vi "Update State Data.vi"(8 "error in (no error)":errorcluster, 9 "Data":variant, 10 "Argument":string, 11 "State Data":T1) -> (0 "error out":errorcluster, 3 "State Data out":T1)   [LabVIEW 2020, in "MacroAssert.lvlib"]
doc: "Updates one or more elements of <B>State Data</B> based on <B>Argument</B> and <B>Data</B>."
uses:
  MacroAssert.lvlib
  CTLs/State Data.ctl
  Classes/Macro/Macro.lvclass
  CTLs/Refs.ctl
  CTLs/Report Data.ctl
  CTLs/Config.ctl
  <vilib>/Utility/error.llb/Error Cluster From Error Code.vi
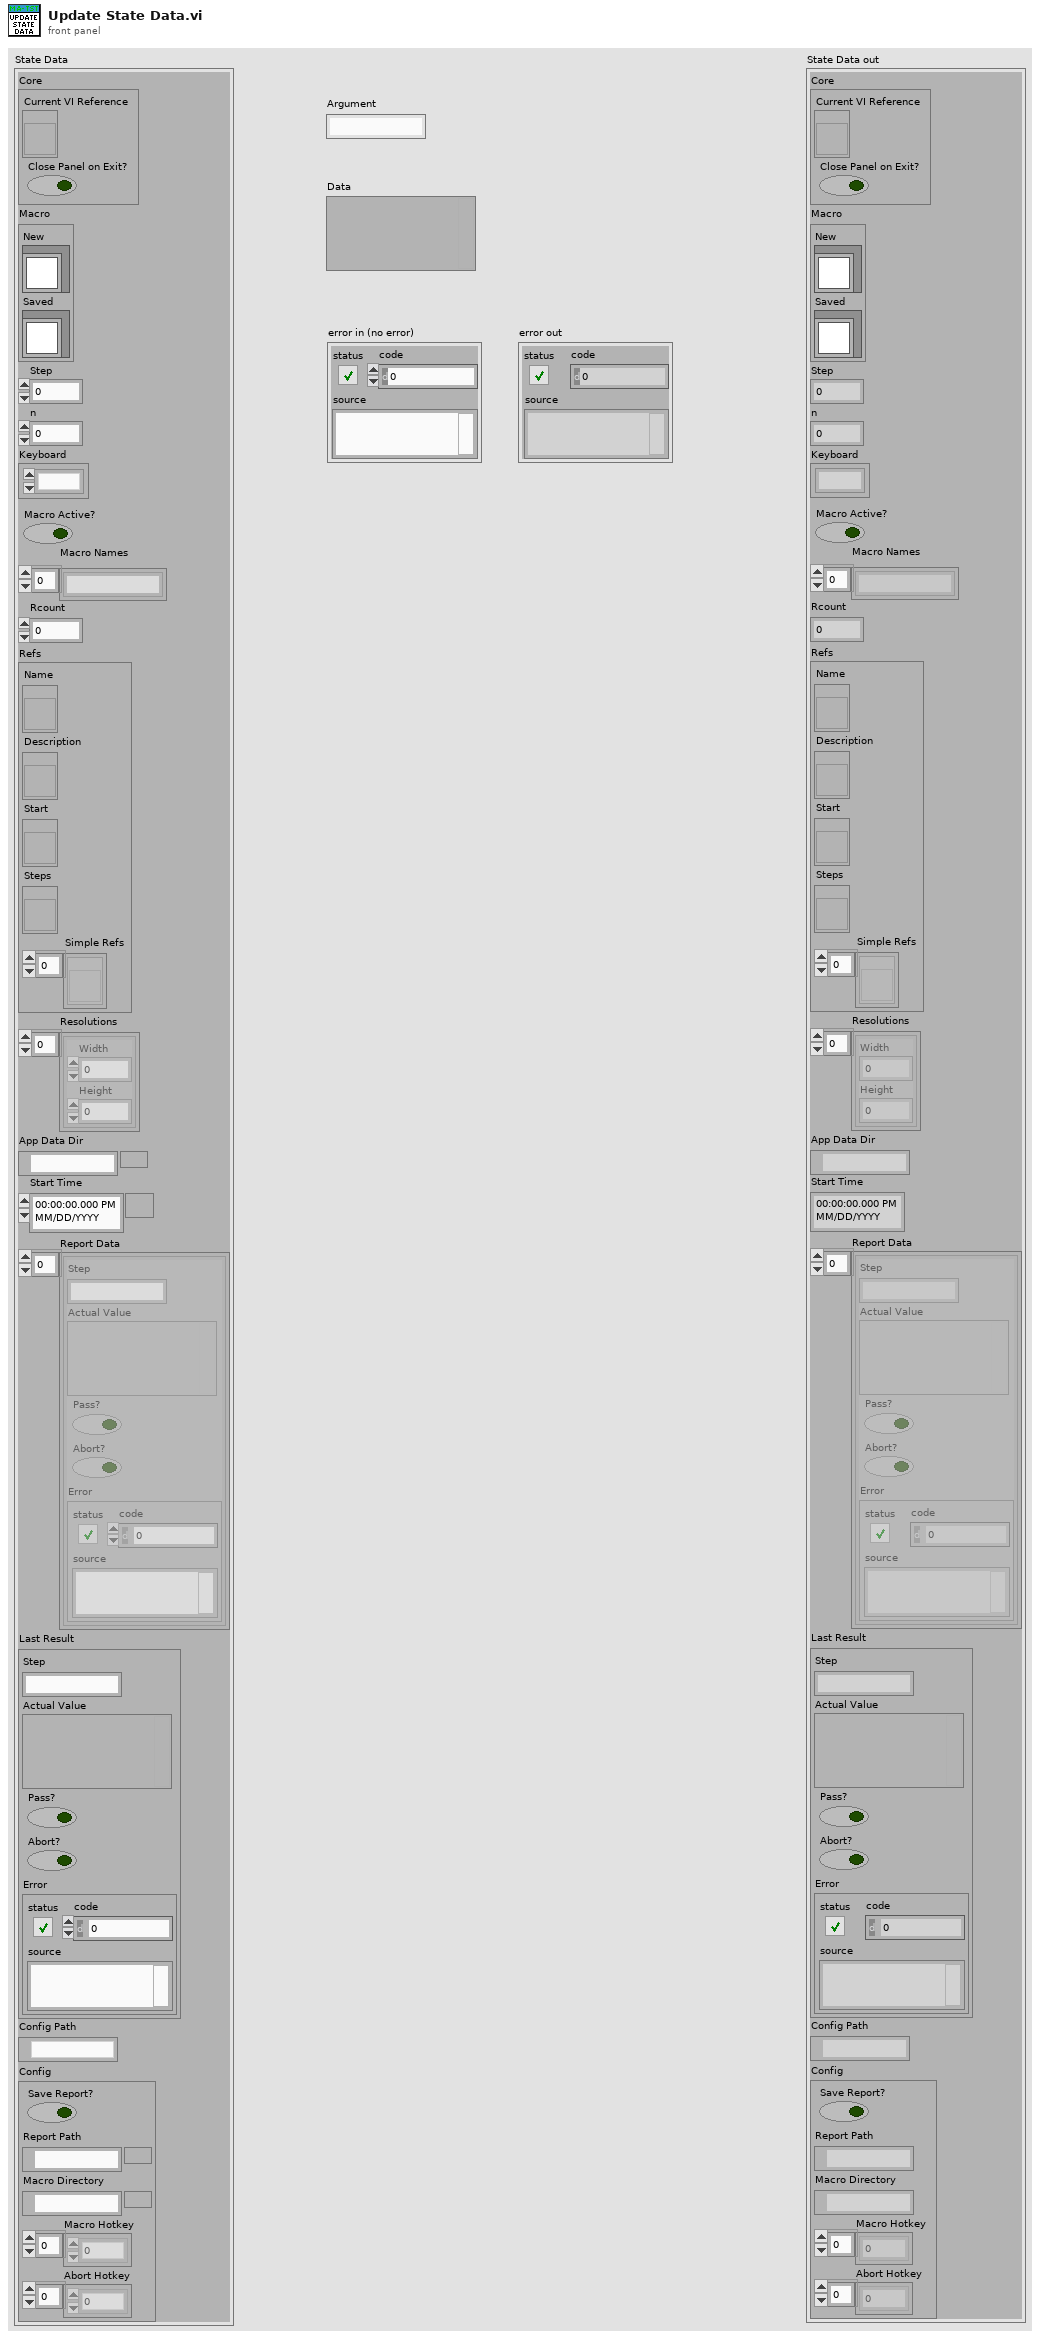
[diagram p1: front panel]
types:
  T1 = typedef "MacroAssert.lvlib/State Data.ctl" = cluster{"Core":cluster{"Current VI Reference":refnum<vi>, "Close Panel on Exit?":bool}, "Macro":cluster{"New":refnum<class "Macro.lvclass">, "Saved":refnum<class "Macro.lvclass">}, "Step":i32, "n":i32, "Keyboard":refnum<k1>, "Macro Active?":bool, "Macro Names":string[], "Rcount":i32, "Refs":T2, "Resolutions":cluster{"Width":i16, "Height":i16}[], "App Data Dir":path, "Start Time":timestamp, "Report Data":T3[], "Last Result":T3, "Config Path":path, "Config":T4}
  T2 = typedef "MacroAssert.lvlib/Refs.ctl" = cluster{"Name":refnum<vi>, "Description":refnum<vi>, "Start":refnum<vi>, "Steps":refnum<vi>, "Simple Refs":refnum<vi>[]}
  T3 = typedef "MacroAssert.lvlib/Report Data.ctl" = cluster{"Step":string, "Actual Value":variant, "Pass?":bool, "Abort?":bool, "Error":errorcluster}
  T4 = typedef "MacroAssert.lvlib/Config.ctl" = cluster{"Save Report?":bool, "Report Path":path, "Macro Directory":path, "Macro Hotkey":enum16{"0", "1", "2", "3", "4", "5", "6", "7", "8", "9", "A", "B", "C", "D", "E", "F", "G", "H", "I", "J", "K", "L", "M", "N", "O", "P", "Q", "R", "S", "T", "U", "V", "W", "X", "Y", "Z", "F1", "F2", "F3", "F4", "F5", "F6", "F7", "F8", "F9", "F10", "F11", "F12", "F13", "F14", "F15", "ADD", "BACK", "BACKSLASH", "CAPITAL", "COMMA", "DECIMAL", "DELETE", "DIVIDE", "DOWN", "END", "EQUALS", "ESCAPE", "GRAVE (`)", "HOME", "INSERT", "LBRACKET", "LCONTROL", "LEFT", "L ALT", "LSHIFT", "LWIN", "MINUS", "MULTIPLY", "NEXT", "NUMLOCK", "NUMPAD_0", "NUMPAD_1", "NUMPAD_2", "NUMPAD_3", "NUMPAD_4", "NUMPAD_5", "NUMPAD_6", "NUMPAD_7", "NUMPAD_8", "NUMPAD_9", "PAUSE", "PERIOD", "PRIOR (PG UP)", "RBRACKET", "RCONTROL", "RETURN", "RIGHT", "R ALT", "RSHIFT", "RWIN", "SCROLL", "SEMICOLON", "SLASH", "SPACE", "SUBTRACT", "TAB", "UP", "ENTER (num pad)", "' (quote)"}[], "Abort Hotkey":enum16{"0", "1", "2", "3", "4", "5", "6", "7", "8", "9", "A", "B", "C", "D", "E", "F", "G", "H", "I", "J", "K", "L", "M", "N", "O", "P", "Q", "R", "S", "T", "U", "V", "W", "X", "Y", "Z", "F1", "F2", "F3", "F4", "F5", "F6", "F7", "F8", "F9", "F10", "F11", "F12", "F13", "F14", "F15", "ADD", "BACK", "BACKSLASH", "CAPITAL", "COMMA", "DECIMAL", "DELETE", "DIVIDE", "DOWN", "END", "EQUALS", "ESCAPE", "GRAVE (`)", "HOME", "INSERT", "LBRACKET", "LCONTROL", "LEFT", "L ALT", "LSHIFT", "LWIN", "MINUS", "MULTIPLY", "NEXT", "NUMLOCK", "NUMPAD_0", "NUMPAD_1", "NUMPAD_2", "NUMPAD_3", "NUMPAD_4", "NUMPAD_5", "NUMPAD_6", "NUMPAD_7", "NUMPAD_8", "NUMPAD_9", "PAUSE", "PERIOD", "PRIOR (PG UP)", "RBRACKET", "RCONTROL", "RETURN", "RIGHT", "R ALT", "RSHIFT", "RWIN", "SCROLL", "SEMICOLON", "SLASH", "SPACE", "SUBTRACT", "TAB", "UP", "ENTER (num pad)", "' (quote)"}[]}
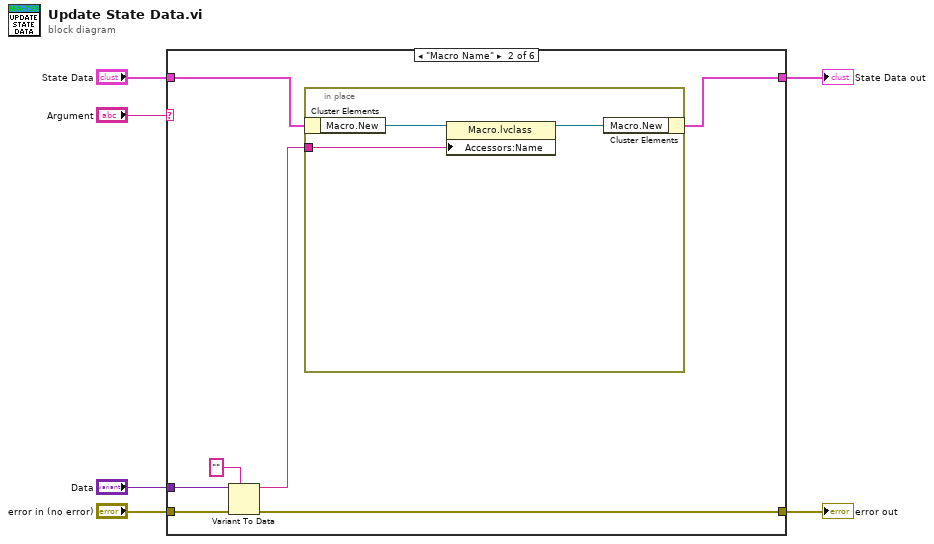
[diagram p0: block diagram]
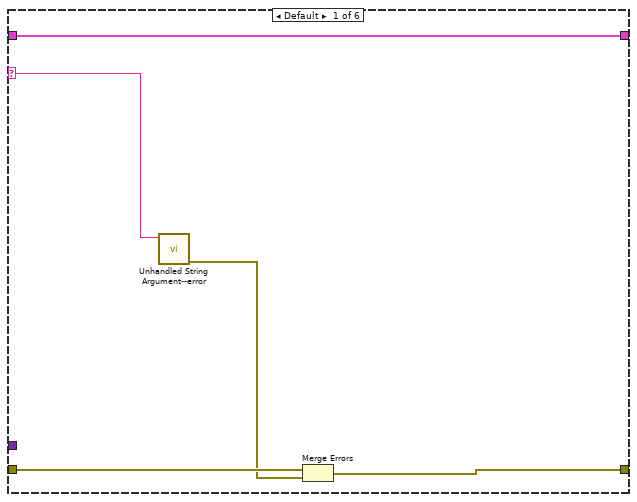
[diagram p2: hidden frame]
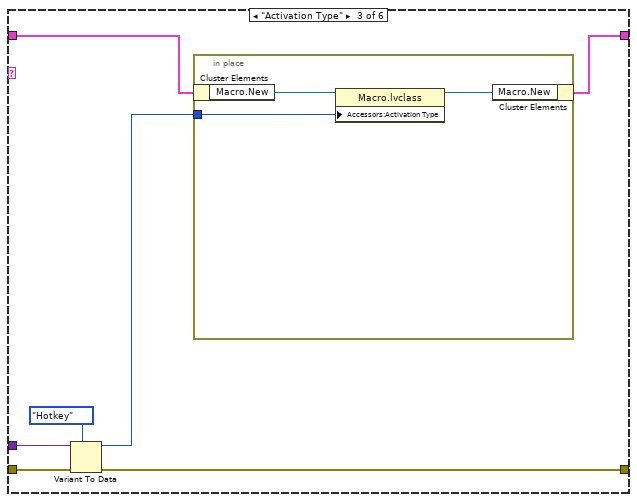
[diagram p3: hidden frame]
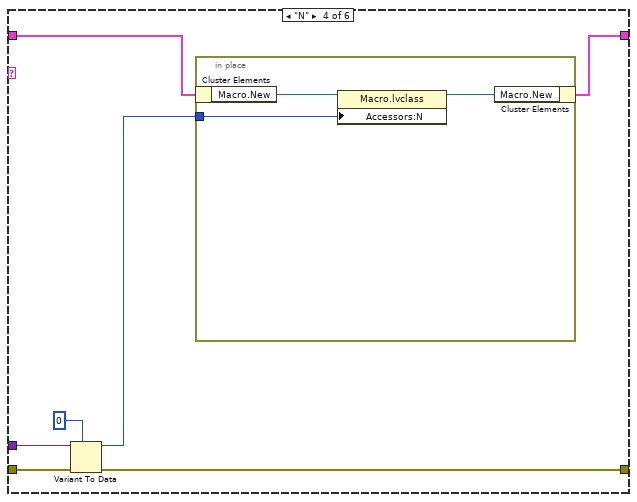
[diagram p4: hidden frame]
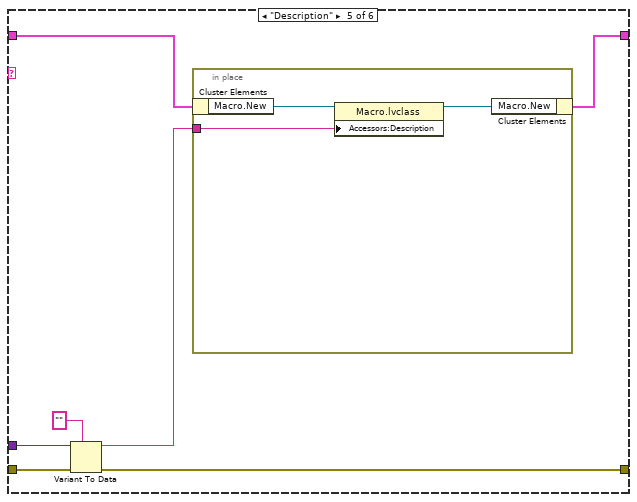
[diagram p5: hidden frame]
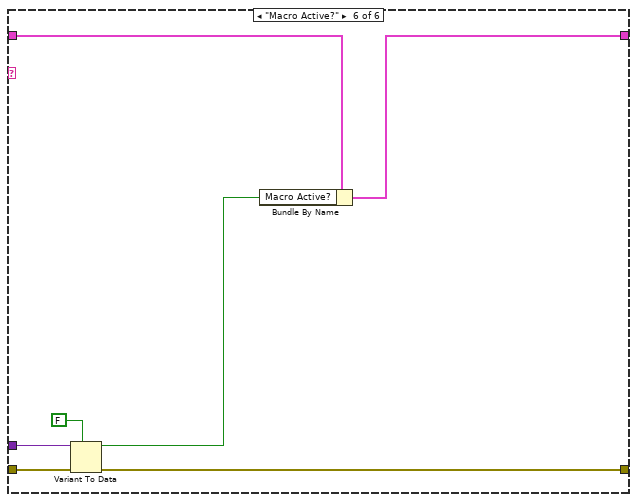
[diagram p6: hidden frame]
diagram:
  n1 = case shown="\"Macro Name\"" "Argument" {
    selector: "Argument" -> [w7 _ _ _ _ _]
    tunnel: "State Data" -> [w10 w14 w24 w34 w43 w55]
    tunnel: "error in (no error)" -> [w11 w18 w28 w38 w48 w58]
    tunnel: "Data" -> [_ w17 w27 w37 w47 w57]
    tunnel: [w10 w13 w23 w33 w44 w54] -> w2
    tunnel: [w9 w15 w26 w36 w46 w53] -> w1
    frame Default {
      n2 = call "Unhandled String Argument--error.vi"("Argument"=w7) -> ("error out"=w8:errorcluster)  [unwired: 10 in]
      n3 = Merge Errors(w11, w8) -> (w9:errorcluster)
    }
    frame "Macro Name" {
      n4 = Variant To Data(error in=w18, type="", Variant=w17) -> (data=w12:string, error out=w15:errorcluster)
      n5 = in-place {
        in-place-border: w12 -> [w19]
        n6 = in-place-cluster #1(w14) -> ("Macro.New"=w21:refnum<class "Macro.lvclass">)
        n7 = property class="Macro.lvclass"(reference=w21, "Accessors:Name"=w19) -> (reference out=w20:refnum<class "Macro.lvclass">)  [unwired: 1 in, 1 out]
        n8 = in-place-cluster #1("Macro.New"=w20) -> (w13:T1)
      }
    }
    frame "Activation Type" {
      n9 = Variant To Data(error in=w28, type=enum32{"Hotkey", "Automatic"}."Hotkey" ("FP CTLs.Type"), Variant=w27) -> (data=w22:enum32{"Hotkey", "Automatic"}, error out=w26:errorcluster)
      n10 = in-place {
        in-place-border: w22 -> [w29]
        n11 = in-place-cluster #2(w24) -> ("Macro.New"=w31:refnum<class "Macro.lvclass">)
        n12 = property class="Macro.lvclass"(reference=w31, "Accessors:Activation Type"=w29) -> (reference out=w30:refnum<class "Macro.lvclass">)  [unwired: 1 in, 1 out]
        n13 = in-place-cluster #2("Macro.New"=w30) -> (w23:T1)
      }
    }
    frame "N" {
      n14 = Variant To Data(error in=w38, type=0 ("FP CTLs.N"), Variant=w37) -> (data=w32:i32, error out=w36:errorcluster)
      n15 = in-place {
        in-place-border: w32 -> [w39]
        n16 = in-place-cluster #3(w34) -> ("Macro.New"=w41:refnum<class "Macro.lvclass">)
        n17 = property class="Macro.lvclass"(reference=w41, "Accessors:N"=w39) -> (reference out=w40:refnum<class "Macro.lvclass">)  [unwired: 1 in, 1 out]
        n18 = in-place-cluster #3("Macro.New"=w40) -> (w33:T1)
      }
    }
    frame "Description" {
      n19 = Variant To Data(error in=w48, type="" ("FP CTLs.N"), Variant=w47) -> (data=w42:string, error out=w46:errorcluster)
      n20 = in-place {
        in-place-border: w42 -> [w49]
        n21 = in-place-cluster #4(w43) -> ("Macro.New"=w51:refnum<class "Macro.lvclass">)
        n22 = property class="Macro.lvclass"(reference=w51, "Accessors:Description"=w49) -> (reference out=w50:refnum<class "Macro.lvclass">)  [unwired: 1 in, 1 out]
        n23 = in-place-cluster #4("Macro.New"=w50) -> (w44:T1)
      }
    }
    frame "Macro Active?" {
      n24 = Variant To Data(error in=w58, type=FALSE, Variant=w57) -> (data=w56:bool, error out=w53:errorcluster)
      n25 = Bundle By Name(cluster=w55, "Macro Active?"=w56) -> (w54:T1)
    }
  }
  "error out" <- w1
  "State Data out" <- w2
